vi "Error - Log.vi"(8 "error in (no error)":errorcluster, 11 "Error Data":T1) -> (0 "error out":errorcluster)   [LabVIEW 2017]
uses:
  Controls/Error Data.ctl
  Controls/Error Type.ctl
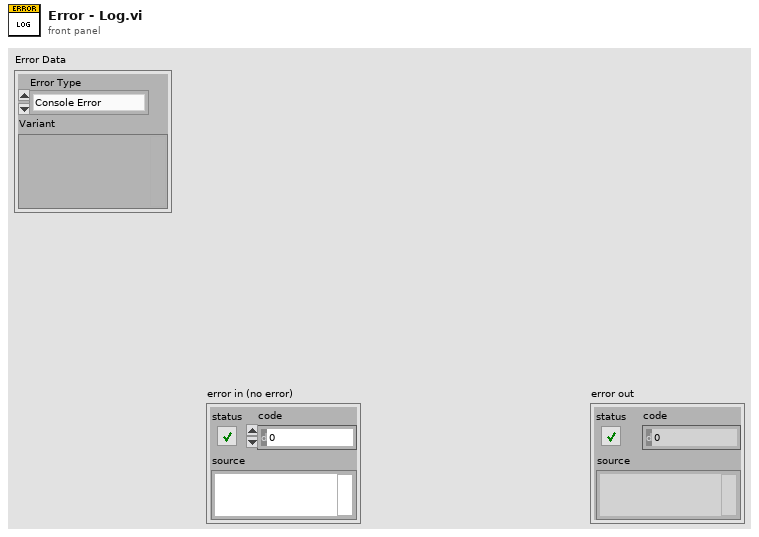
[diagram p1: front panel]
types:
  T1 = typedef "Error Data.ctl" = cluster{"Error Type":T2, "Variant":variant}
  T2 = typedef "Error Type.ctl" = enum16{"Console Error", "Sensor Interface IO Error", "Process Step Error"}
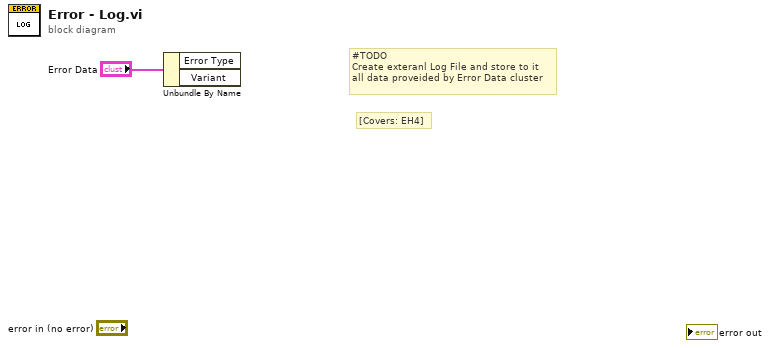
[diagram p0: block diagram]
diagram:
  # "[Covers: EH4]"
  # "#TODO\nCreate exteranl Log File and store to it\nall data proveided by Error Data cluster"
  n1 = Unbundle By Name("Error Data") -> ()  [unwired: 2 out]
